vi "Write Value.vi"(8 "error in (no error)":errorcluster, 10 "value":variant, 11 "NT Scalar in":refnum<class "NT Scalar.lvclass">) -> (0 "error out":errorcluster, 3 "NT Scalar out":refnum<class "NT Scalar.lvclass">)   [LabVIEW 2020, in "PV Access.lvlib" / "PV Data.lvlib" / "NT Scalar.lvclass"]
uses:
  NT Scalar.lvclass
  NT Scalar.lvclass/NT Scalar.ctl
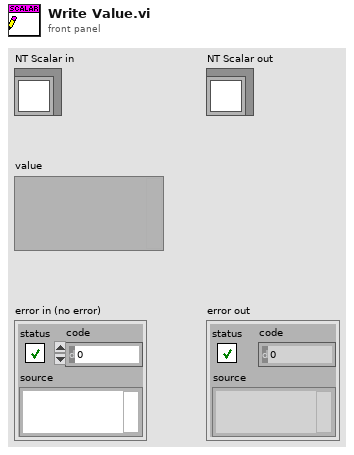
[diagram p1: front panel]
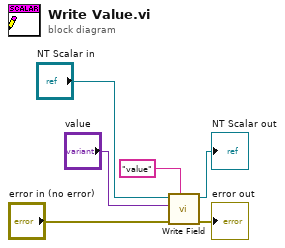
[diagram p0: block diagram]
diagram:
  n1 = call-dynamic "Write Field.vi"("field"="value", "error in (no error)"="error in (no error)", "value"="value", "Base Interface in"="NT Scalar in") -> ("error out"=→"error out":errorcluster, "Base Interface out"=→"NT Scalar out":refnum<class "NT Scalar.lvclass">)  [unwired: 6 in]
